vi "DriveModuleControl_TravTunePID_Report.vi"(3 "Network Table Prefix":string, 5 "TestInProgress":bool, 7 "Tuning Done":bool, 8 "Error Occured":bool, 9 "Diagnostic Info":T2, 10 "Plant and Test Data":T3, 11 "New Tuning Parameters":T1) -> ()   [LabVIEW 2023]
uses:
  <vilib>/Rock Robotics/Network Tables/NT Write Boolean.vi
  <vilib>/Rock Robotics/Network Tables/NT Write Number.vi
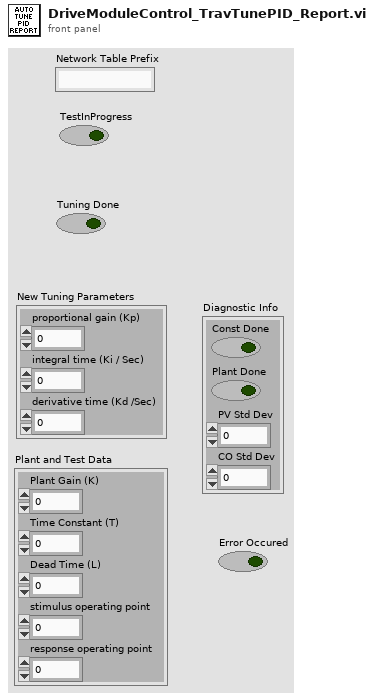
[diagram p1: front panel]
types:
  T1 = cluster{"proportional gain (Kp)":dbl, "integral time (Ki / Sec)":dbl, "derivative time (Kd /Sec)":dbl}
  T2 = cluster{"Const Done":bool, "Plant Done":bool, "PV Std Dev":dbl, "CO Std Dev":dbl}
  T3 = cluster{"Plant Gain (K)":dbl, "Time Constant (T)":dbl, "Dead Time (L)":dbl, "stimulus operating point":dbl, "response operating point":dbl}
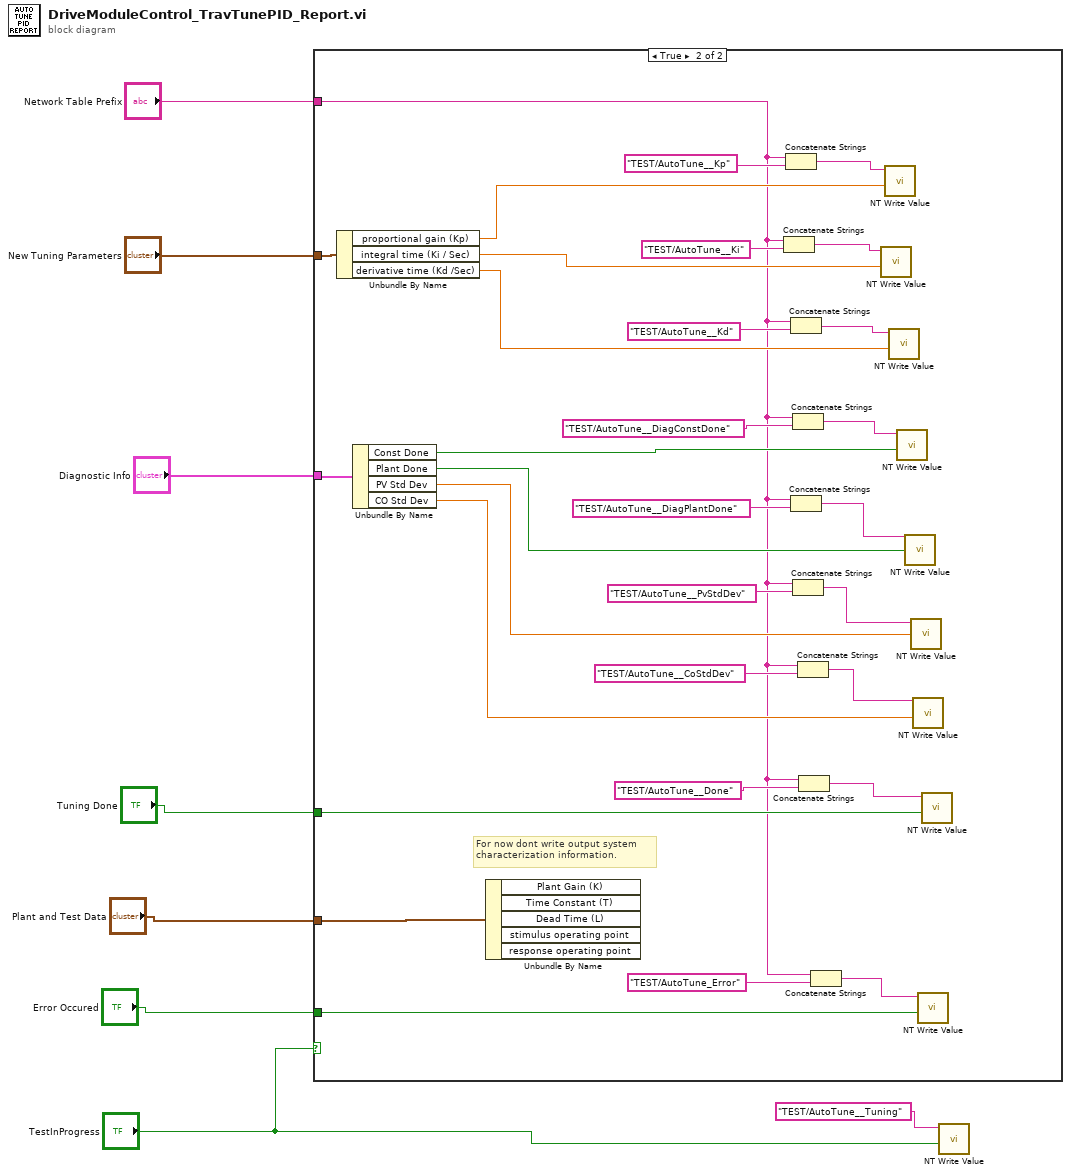
[diagram p0: block diagram]
diagram:
  n1 = case shown="True" "TestInProgress" {
    tunnel: "Network Table Prefix" -> [_ w11]
    tunnel: "Diagnostic Info" -> [_ w25]
    tunnel: "New Tuning Parameters" -> [_ w24]
    tunnel: "Tuning Done" -> [_ w16]
    tunnel: "Plant and Test Data" -> [_ w15]
    tunnel: "Error Occured" -> [_ w14]
    frame False {
    }
    frame True {
      # "For now dont write output system\ncharacterization information."
      n2 = Unbundle By Name(w24) -> ("proportional gain (Kp)"=w17:dbl, "integral time (Ki / Sec)"=w18:dbl, "derivative time (Kd /Sec)"=w19:dbl)
      n3 = Unbundle By Name(w25) -> ("Const Done"=w20:bool, "Plant Done"=w21:bool, "PV Std Dev"=w22:dbl, "CO Std Dev"=w23:dbl)
      n4 = Unbundle By Name(w15) -> ()  [unwired: 5 out]
      n5 = Concatenate Strings(w11, "TEST/AutoTune__Ki" ("name")) -> (w30:string)
      n6 = Concatenate Strings(w11, "TEST/AutoTune__Kp" ("name")) -> (w29:string)
      n7 = Concatenate Strings(w11, "TEST/AutoTune__Kd" ("name")) -> (w31:string)
      n8 = Concatenate Strings(w11, "TEST/AutoTune__DiagPlantDone" ("name")) -> (w37:string)
      n9 = Concatenate Strings(w11, "TEST/AutoTune__DiagConstDone" ("name")) -> (w33:string)
      n10 = Concatenate Strings(w11, "TEST/AutoTune__PvStdDev" ("name")) -> (w38:string)
      n11 = Concatenate Strings(w11, "TEST/AutoTune__CoStdDev" ("name")) -> (w39:string)
      n12 = Concatenate Strings(w11, "TEST/AutoTune__Done" ("name")) -> (w10:string)
      n13 = Concatenate Strings(w11, "TEST/AutoTune_Error" ("name")) -> (w9:string)
      n14 = call-poly <vilib>:"NT Write Value.vi"("value"=w18, "name"=w30) -> ()  [unwired: 9 in, 1 out]
      n15 = call-poly <vilib>:"NT Write Value.vi"("value"=w17, "name"=w29) -> ()  [unwired: 9 in, 1 out]
      n16 = call-poly <vilib>:"NT Write Value.vi"("value"=w19, "name"=w31) -> ()  [unwired: 9 in, 1 out]
      n17 = call-poly <vilib>:"NT Write Value.vi"("value"=w20, "name"=w33) -> ()  [unwired: 9 in, 1 out]
      n18 = call-poly <vilib>:"NT Write Value.vi"("value"=w21, "name"=w37) -> ()  [unwired: 9 in, 1 out]
      n19 = call-poly <vilib>:"NT Write Value.vi"("value"=w22, "name"=w38) -> ()  [unwired: 9 in, 1 out]
      n20 = call-poly <vilib>:"NT Write Value.vi"("value"=w23, "name"=w39) -> ()  [unwired: 9 in, 1 out]
      n21 = call-poly <vilib>:"NT Write Value.vi"("value"=w14, "name"=w9) -> ()  [unwired: 9 in, 1 out]
      n22 = call-poly <vilib>:"NT Write Value.vi"("value"=w16, "name"=w10) -> ()  [unwired: 9 in, 1 out]
    }
  }
  n23 = call-poly <vilib>:"NT Write Value.vi"("value"="TestInProgress", "name"="TEST/AutoTune__Tuning") -> ()  [unwired: 9 in, 1 out]
